vi "AI Loop.vi"() -> ()   [LabVIEW 2012]
uses:
  <vilib>/Platform/TimedLoop/XDataNode/timing_clust.ctl
  <vilib>/Platform/TimedLoop/XDataNode/nitl_modes.ctl
  <vilib>/Platform/TimedLoop/XDataNode/wakeup.ctl
  Utilities/Robot Parameters/Robot Parameters.vi
  <vilib>/Platform/TimedLoop/XDataNode/XDataNode.xnode
  <vilib>/Platform/TimedLoop/XDataNode/XDNodeRunTimeDep.lvlib
panel:
  out "output cluster":T1
  in  "SubGoalOrt":dbl[](array[numeric])
  in  "Direction":dbl[](array[numeric])
  in  "Magnitude":dbl[](array[numeric])
  in  "Line Data":T2(array[cluster])
  out "Outer threshold":dbl
  out "Inner threshold":dbl
  in  "Max speed (m/s)":dbl=0.5
  in  "No Occupancy":bool=TRUE
  out "Heading_Cmd":dbl
  out "VTan_Cmd":dbl
  out "VAng_Cmd":dbl
  out "Error Out":errorcluster
  in  "Error In":errorcluster
  in  "stop?":bool
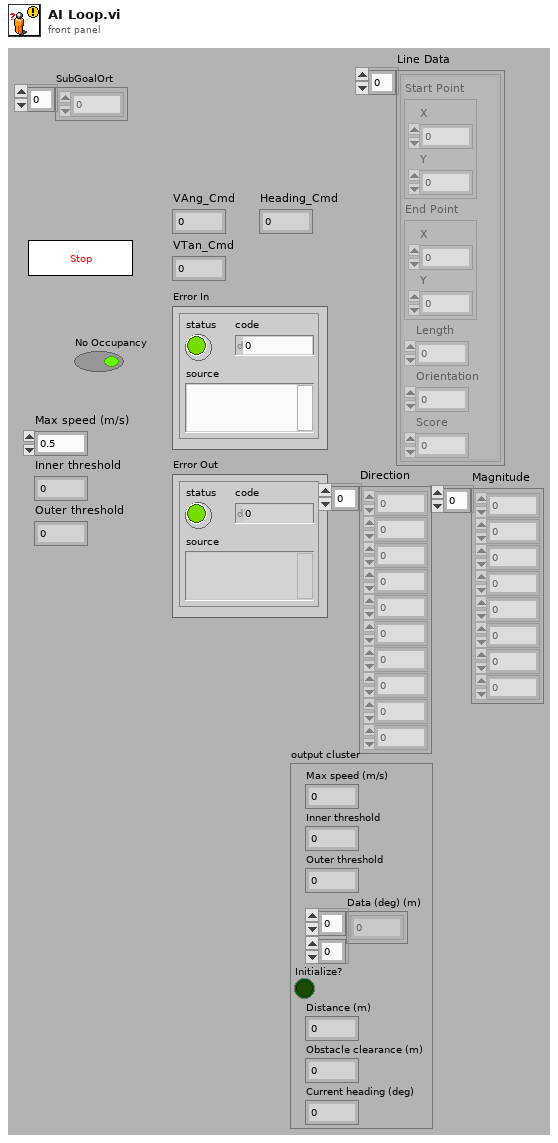
[diagram p1: front panel]
types:
  T1 = cluster{"Max speed (m/s)":dbl, "Inner threshold":dbl, "Outer threshold":dbl, "Data (deg) (m)":dbl[][], "Initialize?":bool, "Distance (m)":dbl, "Obstacle clearance (m)":dbl, "Current heading (deg)":dbl}
  T2 = cluster{"Start Point":cluster{"X":sgl, "Y":sgl}, "End Point":cluster{"X":sgl, "Y":sgl}, "Length":dbl, "Orientation":dbl, "Score":dbl}[]
  T3 = enum16{"Idle", "Wiimote", "Joypad", "IGVC", "Avoide Objects", "Avoide Lines", "Path Planning", "Heading", "Waypoint"}
  T4 = typedef "XDNodeRunTimeDep.lvlib/timing_clust.ctl" = cluster{"Expected End [f-1]":u64, "Actual End [f-1]":u64, "Finished Late? [f-1]":bool, "Expected End [i-1]":u64, "Actual End [i-1]":u64, "Finished Late? [i-1]":bool, "Expected Start [i]":u64, "Actual Start [i]":u64, "Expected Start [f]":u64, "Actual Start [f]":u64, "Source Name":string, "Structure Name":string, "Period":i64, "Deadline":i64, "Offset":i64, "Start":i64, "Priority":i32, "Timeout":i32, "Mode":T5, "Wakeup Reason":T6, "Error":errorcluster, "Source Type":string, "Secondary Source Type":string, "Global End Time":u64, "Global Start Time":u64, "Frame Duration":u64, "Iteration Duration":u64, "Assigned CPU":i32, "I/O Scan Engine Mode":u32}
  T5 = typedef "XDNodeRunTimeDep.lvlib/nitl_modes.ctl" = enum32{"No Change", "Process missed periods, maintain original phase", "Discard missed periods, maintain original phase", "Process missed periods, ignore original phase", "Discard missed periods, ignore original phase"}
  T6 = typedef "XDNodeRunTimeDep.lvlib/wakeup.ctl" = enum32{"Normal", "Aborted", "Asynchronous wakeup", "Timing source error", "Timed loop error", "Timeout"}
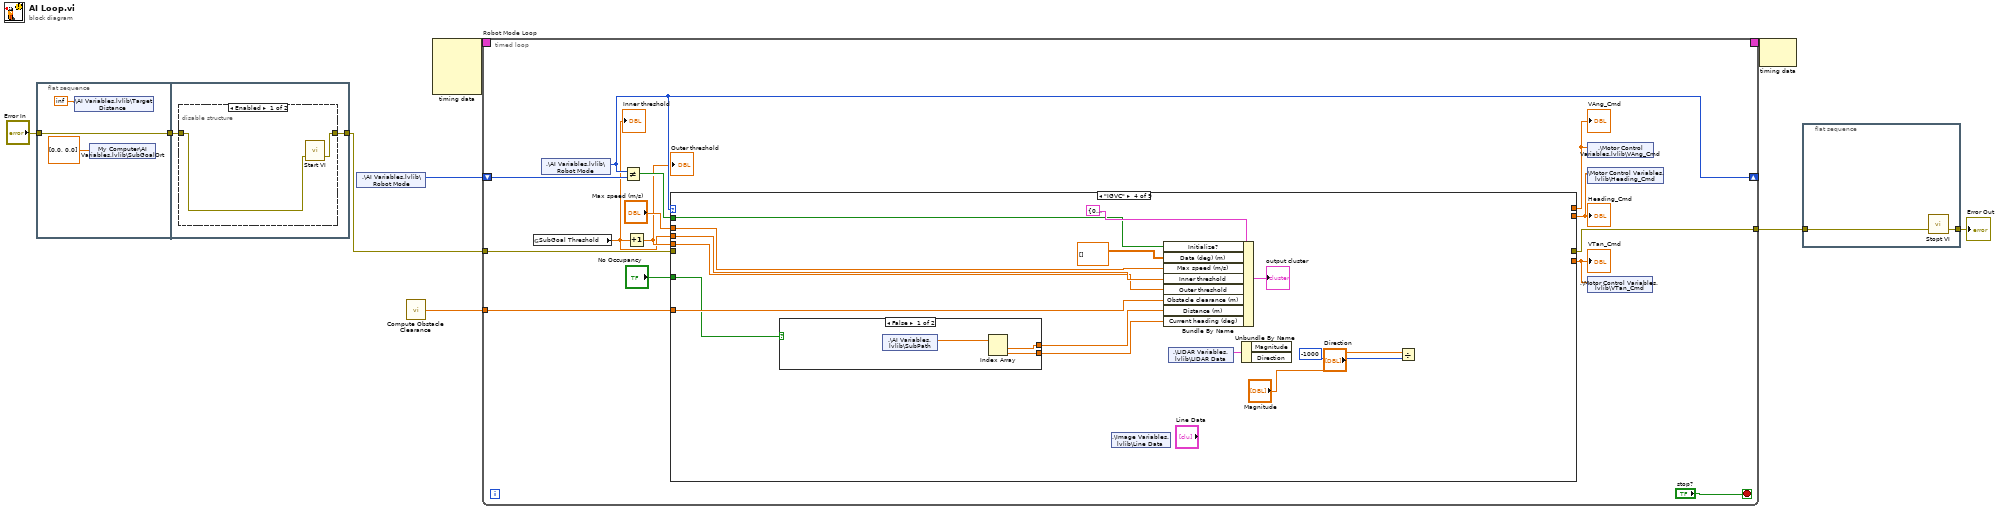
[diagram p0: block diagram]
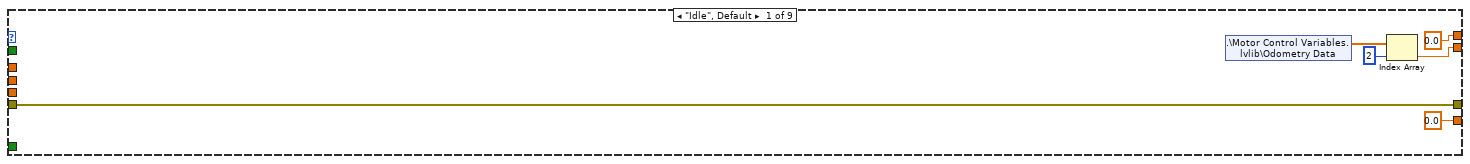
[diagram p3: hidden frame]
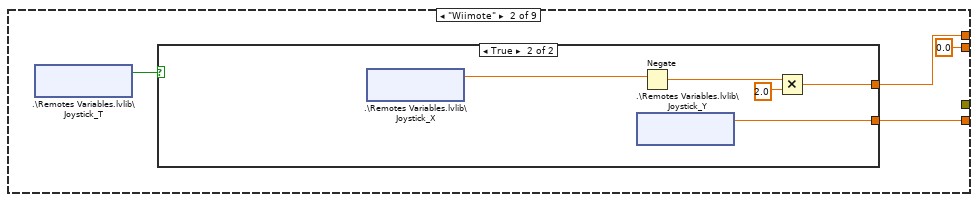
[diagram p4: hidden frame]
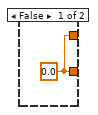
[diagram p5: hidden frame]
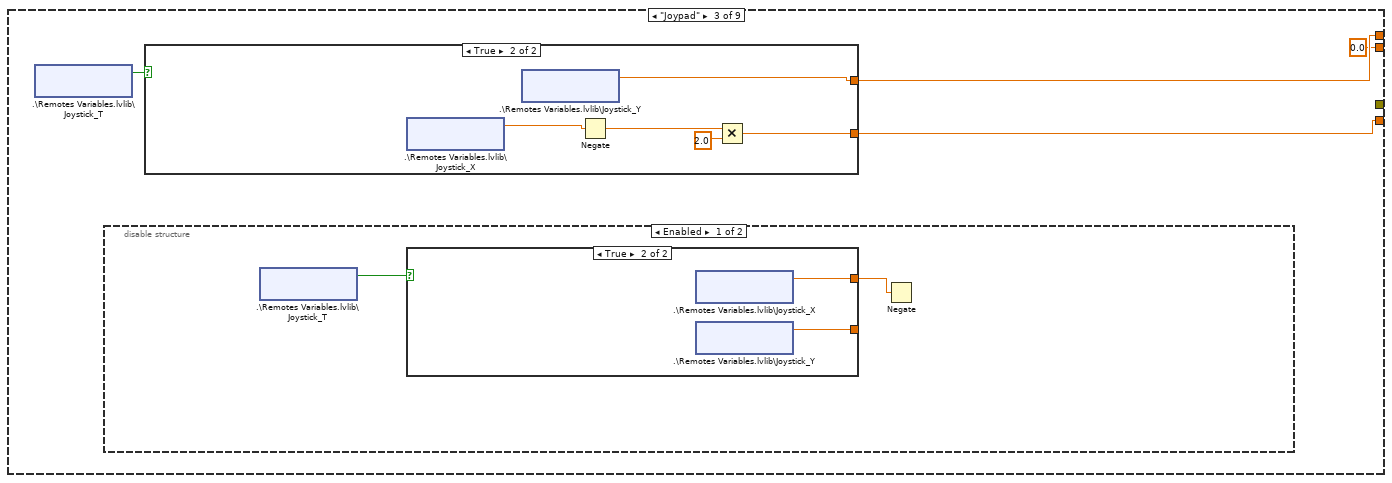
[diagram p6: hidden frame]
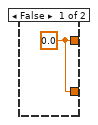
[diagram p7: hidden frame]
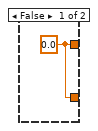
[diagram p9: hidden frame]
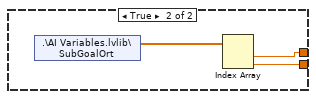
[diagram p10: hidden frame]
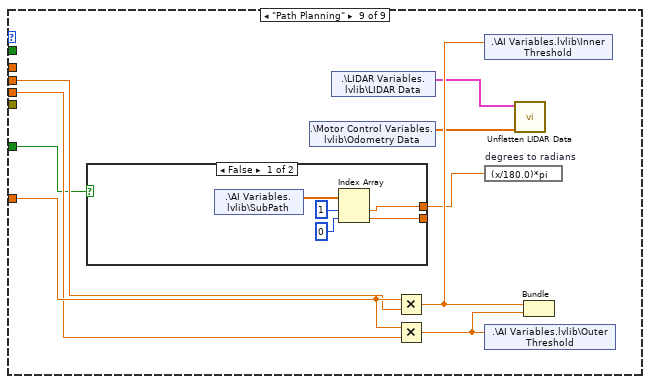
[diagram p15: hidden frame]
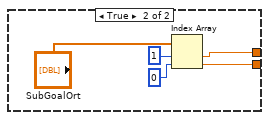
[diagram p16: hidden frame]
diagram:
  n1 = flat-sequence {
    tunnel: "Error In" -> [w11]
    tunnel: [w11] -> w4
    tunnel: [w13] -> w5
    tunnel: w4 -> [w14]
    frame #0 {
      n2 = shared-variable ".\\AI Variables.lvlib\\Target Distance"(inf) -> ()  [unwired: 1 in, 1 out]
      n3 = shared-variable "My Computer\\AI Variables.lvlib\\SubGoalOrt"(dbl[] [0.0, 0.0] ("SubGoalOrt")) -> ()  [unwired: 1 in, 1 out]
    }
    frame #1 {
      n4 = disable-structure shown="Enabled" {
        disable-tunnel: w14 -> [w16 w17]
        disable-tunnel: [w15 w17] -> w13
        frame Enabled {
          n5 = call "Start VI.vi"("error in"=w16) -> ("error out"=w15:errorcluster)  [unwired: 2 in]
        }
        frame Disabled {
        }
      }
    }
  }
  n6 = shared-variable ".\\AI Variables.lvlib\\Robot Mode"() -> (w7:T3)  [unwired: 1 in, 1 out]
  n7 = call "Compute Obstacle Clearance.vi"() -> ("obstacle clearance (m)"=w1:dbl)  [unwired: 1 in]
  n8 = node-c288() -> (w9:T4)  [unwired: 4 in]
  n9 = timed-loop "Robot Mode Loop" {
    timing: w9 -> [_]
    timing-out: [_] -> w8
    tunnel: w1 -> [w31]
    shift-right: [w28] -> _
    shift-left: w7 -> [w29]
    tunnel: w5 -> [w21]
    tunnel: [w20] -> w2
    stop <- "stop?" stop-if-true
    n10 = global read "Robot Parameters.vi" "SubGoal Threshold"() -> (w18:dbl)
    "Inner threshold" <- w18
    n11 = shared-variable ".\\AI Variables.lvlib\\Robot Mode"() -> (w28:T3)  [unwired: 1 in, 1 out]
    n12 = Not Equal?(x=w28, y=w29) -> (x != y?=w30:bool)
    n13 = Increment(x=w18) -> (x+1=w19:dbl)
    "Outer threshold" <- w19
    n14 = case shown="\"IGVC\"" w28 {
      tunnel: w31 -> [_ _ _ w70 _ _ _ _ w91]
      tunnel: [w33 0.0 ("Numeric") 0.0 ("Numeric") _ _ _ _ _ _] -> w27
      tunnel: [0.0 ("Double") w40 w48 _ _ _ _ _ _] -> w26
      tunnel: [0.0 w39 w50 _ _ _ _ _ _] -> w25
      tunnel: w30 -> [_ _ _ w71 _ _ _ _ _]
      tunnel: w18 -> [_ _ _ w74 _ _ _ _ w85]
      tunnel: w19 -> [_ _ _ w73 _ _ _ _ w84]
      tunnel: "Max speed (m/s)" -> [_ _ _ w75 _ _ _ _ _]
      tunnel: "No Occupancy" -> [_ _ _ w69 _ _ _ _ w83]
      tunnel: w21 -> [w32 _ _ _ _ _ _ _ _]
      tunnel: [w32 _ _ _ _ _ _ _ _] -> w20
      frame "Idle", Default {
        n15 = shared-variable ".\\Motor Control Variables.lvlib\\Odometry Data"() -> (w35:dbl[])  [unwired: 1 in, 1 out]
        n16 = Index Array(array=w35, index=2) -> (element=w33:dbl)
      }
      frame "Wiimote" {
        n17 = shared-variable ".\\Remotes Variables.lvlib\\Joystick_T"() -> (w41:bool)  [unwired: 1 in, 2 out]
        n18 = case shown="True" w41 {
          tunnel: [w42 w44] -> w40
          tunnel: [w42 w46] -> w39
          frame False {
            w42 = 0.0
          }
          frame True {
            n19 = shared-variable ".\\Remotes Variables.lvlib\\Joystick_X"() -> (w43:dbl)  [unwired: 1 in, 2 out]
            n20 = shared-variable ".\\Remotes Variables.lvlib\\Joystick_Y"() -> (w44:dbl)  [unwired: 1 in, 2 out]
            n21 = Negate(x=w43) -> (-x=w47:dbl)
            n22 = Multiply(x=w47, y=2.0) -> (x*y=w46:dbl)
          }
        }
      }
      frame "Joypad" {
        n23 = shared-variable ".\\Remotes Variables.lvlib\\Joystick_T"() -> (w51:bool)  [unwired: 1 in, 2 out]
        n24 = disable-structure shown="Enabled" {
          frame Enabled {
            n25 = shared-variable ".\\Remotes Variables.lvlib\\Joystick_T"() -> (w53:bool)  [unwired: 1 in, 2 out]
            n26 = case shown="True" w53 {
              tunnel: [w54 w55] -> _
              tunnel: [w54 w56] -> w52
              frame False {
                w54 = 0.0
              }
              frame True {
                n27 = shared-variable ".\\Remotes Variables.lvlib\\Joystick_X"() -> (w56:dbl)  [unwired: 1 in, 2 out]
                n28 = shared-variable ".\\Remotes Variables.lvlib\\Joystick_Y"() -> (w55:dbl)  [unwired: 1 in, 2 out]
              }
            }
            n29 = Negate(x=w52) -> ()  [unwired: 1 out]
          }
          frame Disabled {
          }
        }
        n30 = case shown="True" w51 {
          tunnel: [w57 w58] -> w50
          tunnel: [w57 w61] -> w48
          frame False {
            w57 = 0.0
          }
          frame True {
            n31 = shared-variable ".\\Remotes Variables.lvlib\\Joystick_X"() -> (w59:dbl)  [unwired: 1 in, 2 out]
            n32 = shared-variable ".\\Remotes Variables.lvlib\\Joystick_Y"() -> (w58:dbl)  [unwired: 1 in, 2 out]
            n33 = Negate(x=w59) -> (-x=w62:dbl)
            n34 = Multiply(x=w62, y=2.0) -> (x*y=w61:dbl)
          }
        }
      }
      frame "IGVC" {
        n35 = case shown="False" w69 {
          tunnel: [w78 w81] -> w68
          tunnel: [w77 w80] -> w66
          frame False {
            n36 = shared-variable ".\\AI Variables.lvlib\\SubPath"() -> (w79:dbl[])  [unwired: 1 in, 1 out]
            n37 = Index Array(array=w79) -> (element #1=w78:dbl, element #2=w77:dbl)  [unwired: 2 in]
          }
          frame True {
            n38 = shared-variable ".\\AI Variables.lvlib\\SubGoalOrt"() -> (w82:dbl[])  [unwired: 1 in, 1 out]
            n39 = Index Array(array=w82) -> (element #1=w81:dbl, element #2=w80:dbl)  [unwired: 2 in]
          }
        }
        n40 = shared-variable ".\\Image Variables.lvlib\\Line Data"() -> ()  [unwired: 1 in, 2 out]
        n41 = Bundle By Name(cluster=T1 {"Max speed (m/s)"=0.4, "Inner threshold"=0.6, "Outer threshold"=1.1, "Data (deg) (m)"=[], "Initialize?"=FALSE, "Distance (m)"=0.0, "Obstacle clearance (m)"=1.0, "Current heading (deg)"=0.0} ("Control"), "Initialize?"=w71, "Data (deg) (m)"=dbl[][] [], "Max speed (m/s)"=w75, "Inner threshold"=w74, "Outer threshold"=w73, "Obstacle clearance (m)"=w70, "Distance (m)"=w68, "Current heading (deg)"=w66) -> (→"output cluster":T1)
        n42 = shared-variable ".\\LIDAR Variables.lvlib\\LIDAR Data"() -> (w72:cluster{"Magnitude":dbl[], "Direction":dbl[]})  [unwired: 1 in, 1 out]
        n43 = Unbundle By Name(w72) -> ()  [unwired: 2 out]
        n44 = Divide(x="Magnitude", y=-1000) -> ()  [unwired: 1 out]
      }
      frame "Avoide Objects" {
      }
      frame "Avoide Lines" {
      }
      frame "Heading" {
      }
      frame "Waypoint" {
      }
      frame "Path Planning" {
        n45 = case shown="False" w83 {
          tunnel: [w94 w99] -> w86
          tunnel: [w93 w98] -> _
          frame False {
            n46 = shared-variable ".\\AI Variables.lvlib\\SubPath"() -> (w92:dbl[])  [unwired: 1 in, 1 out]
            n47 = Index Array(array=w92, index #1=1 ("index"), index #2=0 ("index")) -> (element #1=w94:dbl, element #2=w93:dbl)
          }
          frame True {
            n48 = Index Array(array="SubGoalOrt", index #1=1 ("index"), index #2=0 ("index")) -> (element #1=w99:dbl, element #2=w98:dbl)
          }
        }
        n49 = shared-variable ".\\Motor Control Variables.lvlib\\Odometry Data"() -> (w87:dbl[])  [unwired: 1 in, 1 out]
        n50 = shared-variable ".\\LIDAR Variables.lvlib\\LIDAR Data"() -> (w88:cluster{"Magnitude":dbl[], "Direction":dbl[]})  [unwired: 1 in, 1 out]
        n51 = Multiply(x=w91, y=w85) -> (x*y=w90:dbl)
        n52 = Multiply(x=w91, y=w84) -> (x*y=w89:dbl)
        n53 = shared-variable ".\\AI Variables.lvlib\\Inner Threshold"(w90) -> ()  [unwired: 1 in, 1 out]
        n54 = expression code="(x/180.0)*pi" "degrees to radians"(w86) -> ()  [unwired: 1 out]
        n55 = shared-variable ".\\AI Variables.lvlib\\Outer Threshold"(w89) -> ()  [unwired: 1 in, 1 out]
        n56 = call "Unflatten LIDAR Data.vi"("Odometry Data"=w87, "LIDAR Data"=w88) -> ()  [unwired: 8 in, 2 out]
        n57 = Bundle(w90, w89) -> ()  [unwired: 1 in, 1 out]
      }
    }
    "VAng_Cmd" <- w25
    "VTan_Cmd" <- w26
    "Heading_Cmd" <- w27
    n58 = shared-variable ".\\Motor Control Variables.lvlib\\VAng_Cmd"(w25) -> ()  [unwired: 1 in, 1 out]
    n59 = shared-variable ".\\Motor Control Variables.lvlib\\Heading_Cmd"(w27) -> ()  [unwired: 1 in, 1 out]
    n60 = shared-variable ".\\Motor Control Variables.lvlib\\VTan_Cmd"(w26) -> ()  [unwired: 1 in, 1 out]
  }
  n61 = node-c288(w8) -> ()  [unwired: 1 out]
  n62 = flat-sequence {
    tunnel: [w104] -> w3
    tunnel: w2 -> [w105]
    frame #0 {
      n63 = call "Stopt VI.vi"("error in"=w105) -> ("error out"=w104:errorcluster)  [unwired: 2 in]
    }
  }
  "Error Out" <- w3
